vi "Climb Joystick.vi"(1 "Driver Left Bumper":bool, 2 "Driver Right Bumper":bool) -> (0 "Climb Teleop Command":T1)   [LabVIEW 2019]
uses:
  Climb Mode Type Def.ctl
  Climb Command Type Def.ctl
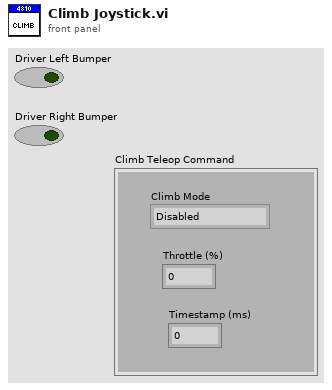
[diagram p1: front panel]
types:
  T1 = typedef "Climb Command Type Def.ctl" = cluster{"Climb Mode":T2, "Throttle (%)":dbl, "Timestamp (ms)":dbl}
  T2 = typedef "Climb Mode Type Def.ctl" = enum16{"Disabled", "Raw Throttle", "Auto Climb"}
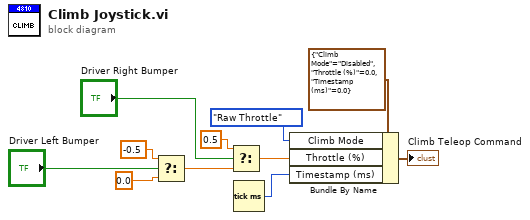
[diagram p0: block diagram]
diagram:
  n1 = Select(t=-0.5, s="Driver Left Bumper", f=0.0) -> (s? t:f=w7:dbl)
  n2 = Select(t=0.5, s="Driver Right Bumper", f=w7) -> (s? t:f=w4:dbl)
  n3 = Tick Count (ms)() -> (millisecond timer value=w2:u32)
  n4 = Bundle By Name(cluster=T1 {"Climb Mode"=enum."Disabled", "Throttle (%)"=0.0, "Timestamp (ms)"=0.0} ("Climb Command"), "Climb Mode"=Climb_Mode_Type_Def."Raw Throttle", "Throttle (%)"=w4, "Timestamp (ms)"=w2) -> (→"Climb Teleop Command":T1)
